vi "multiplier16.vi"(1 "Y":i16, 2 "X":i16) -> (0 "XY":i16)   [LabVIEW 2009]
doc: "Multiplies two I16's. Output is an I16."
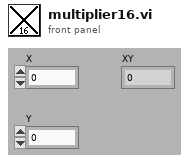
[diagram p1: front panel]
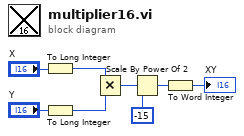
[diagram p0: block diagram]
diagram:
  n1 = To Long Integer(number="X") -> (32bit integer=w5:i32)
  n2 = To Long Integer(number="Y") -> (32bit integer=w3:i32)
  n3 = Multiply(x=w5, y=w3) -> (x*y=w8:i32)
  n4 = Scale By Power Of 2(n=i16 -15, x=w8) -> (x*2^n=w7:i32)
  n5 = To Word Integer(number=w7) -> (16bit integer=→"XY":i16)
